vi "配置文件读取写入.vi"(7 "配置模式":enum16{"读取", "写入"}(ring), 8 "error in (no error)":errorcluster caption="错误输入（无错误）", 10 "配置文件名":string, 11 "配置信息":T6={"周期模式"=enum."不启用", "测量参数"={"氨氮"=TRUE, "总磷"=TRUE, "总氮"=TRUE, "CODMn"=TRUE, "CODCr"=FALSE}, "定点周期"={"启动命令"=enum."", "启动命令 2"=enum."", "启动命令 3"=enum."", "启动命令 4"=enum."", "启动命令 5"=enum."", "启动命令 6"=enum."", "启动命令 7"=enum."", "启动命令 8"=enum."", "启动命令 9"=enum."", "启动命令 10"=enum."", "启动命令 11"=enum."", "启动命令 12"=enum."", "启动命令 13"=enum."", "启动命令 14"=enum."", "启动命令 15"=enum."", "启动命令 16"=enum."", "启动命令 17"=enum."", "启动命令 18"=enum."", "启动命令 19"=enum."", "启动命令 20"=enum."", "启动命令 21"=enum."", "启动命令 22"=enum."", "启动命令 23"=enum."", "启动命令 24"=enum.""}, "间隔启动"={"启动命令"=enum."", "启动间隔"=0.0, "启动次数"=0}}) -> (0 "error out":errorcluster caption="错误输出", 3 "配置信息读取":T6={"周期模式"=enum."不启用", "测量参数"={"氨氮"=TRUE, "总磷"=TRUE, "总氮"=TRUE, "CODMn"=TRUE, "CODCr"=FALSE}, "定点周期"={"启动命令"=enum."", "启动命令 2"=enum."", "启动命令 3"=enum."", "启动命令 4"=enum."", "启动命令 5"=enum."", "启动命令 6"=enum."", "启动命令 7"=enum."", "启动命令 8"=enum."", "启动命令 9"=enum."", "启动命令 10"=enum."", "启动命令 11"=enum."", "启动命令 12"=enum."", "启动命令 13"=enum."", "启动命令 14"=enum."", "启动命令 15"=enum."", "启动命令 16"=enum."", "启动命令 17"=enum."", "启动命令 18"=enum."", "启动命令 19"=enum."", "启动命令 20"=enum."", "启动命令 21"=enum."", "启动命令 22"=enum."", "启动命令 23"=enum."", "启动命令 24"=enum.""}, "间隔启动"={"启动命令"=enum."", "启动间隔"=0.0, "启动次数"=0}})   [LabVIEW 2016, in "ZK定时设置.xctl"]
uses:
  <vilib>/Utility/xml.llb/Read From XML File(string).vi
  <vilib>/Utility/xml.llb/Write to XML File(string).vi
panel:
  # "分钟"
  # "次"
  # "分钟"
  # "次"
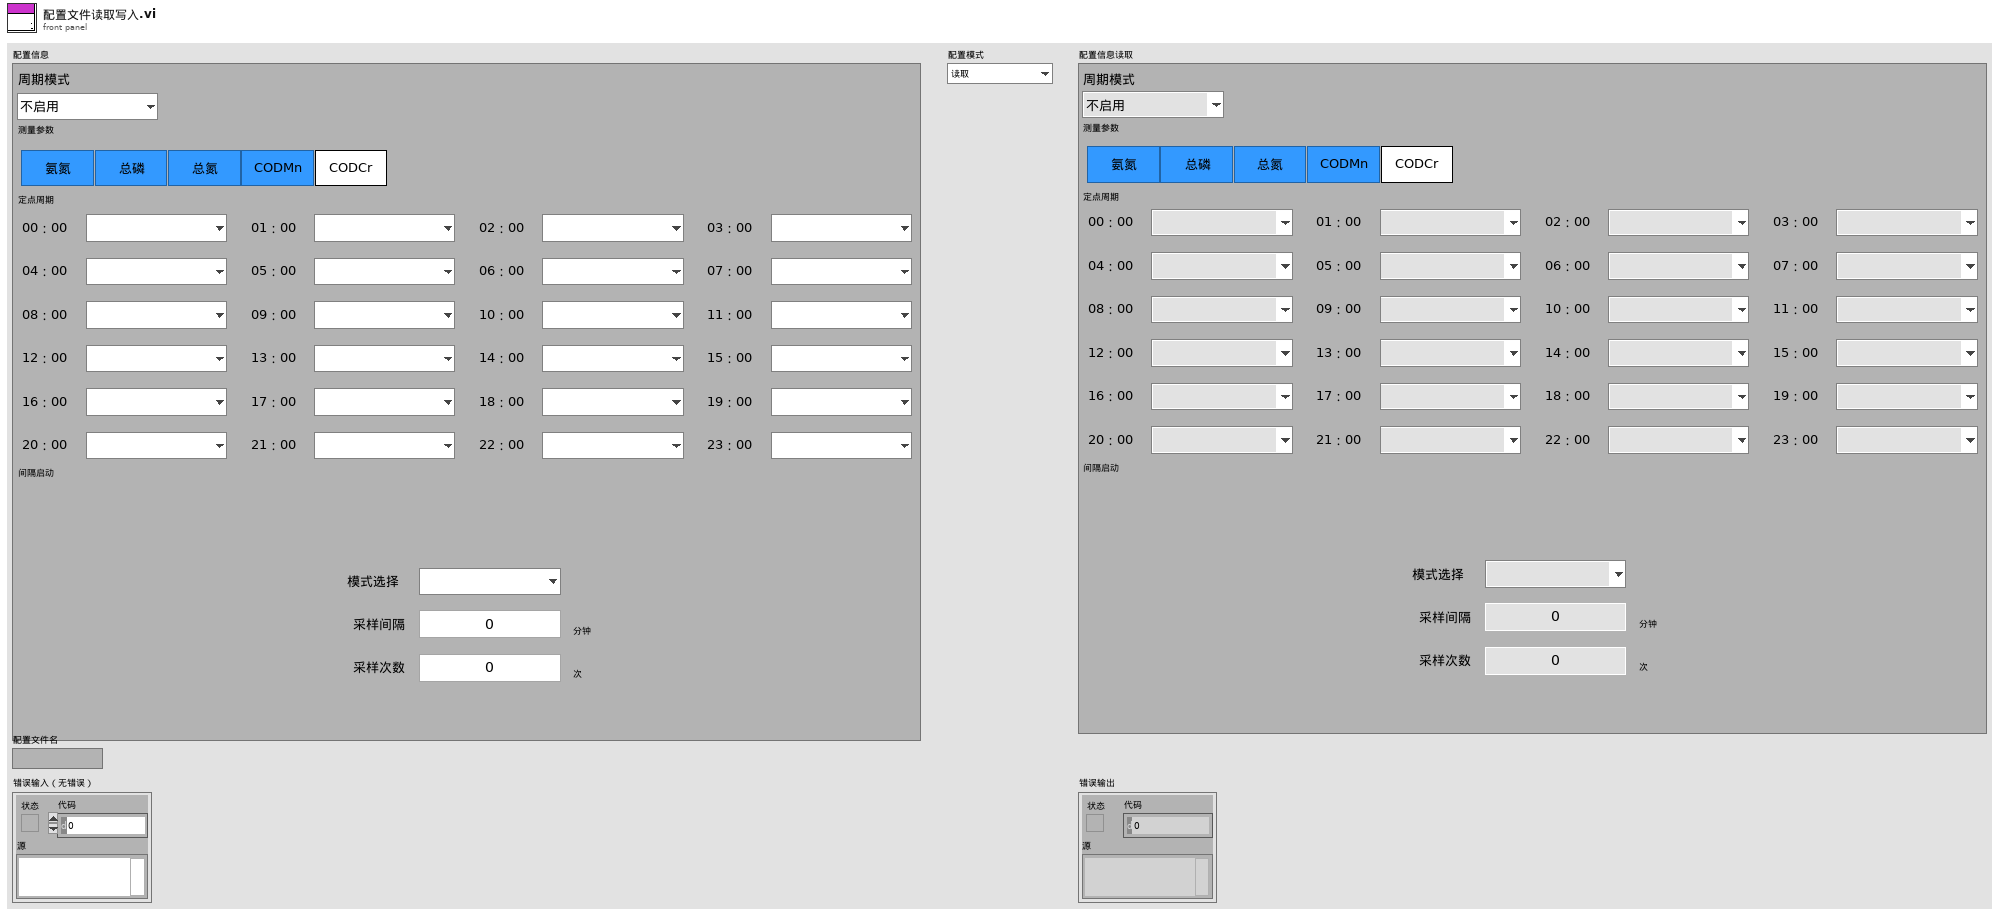
[diagram p1: front panel]
types:
  T1 = typedef "ZK定时设置.xctl/周期模式设置.ctl" = enum16{"不启用", "定点模式", "间隔模式"}
  T2 = typedef "ZK定时设置.xctl/测量参数.ctl" = cluster{"氨氮":bool, "总磷":bool, "总氮":bool, "CODMn":bool, "CODCr":bool}
  T3 = typedef "ZK定时设置.xctl/定点周期设置.ctl" = cluster{"启动命令":T4, "启动命令 2":T4, "启动命令 3":T4, "启动命令 4":T4, "启动命令 5":T4, "启动命令 6":T4, "启动命令 7":T4, "启动命令 8":T4, "启动命令 9":T4, "启动命令 10":T4, "启动命令 11":T4, "启动命令 12":T4, "启动命令 13":T4, "启动命令 14":T4, "启动命令 15":T4, "启动命令 16":T4, "启动命令 17":T4, "启动命令 18":T4, "启动命令 19":T4, "启动命令 20":T4, "启动命令 21":T4, "启动命令 22":T4, "启动命令 23":T4, "启动命令 24":T4}
  T4 = typedef "ZK定时设置.xctl/启动命令选择.ctl" = enum16{"", "加标回收（启动采配水）", "加标回收（不启动采配水）", "水样测试（启动采配水）", "水样测试（不启动采配水）", "平行样测试（启动采配水）", "平行样测试（不启动采配水）", "集成干预测试"}
  T5 = typedef "ZK定时设置.xctl/间隔启动设置.ctl" = cluster{"启动命令":T4, "启动间隔":dbl, "启动次数":i32}
  T6 = cluster{"周期模式":T1, "测量参数":T2, "定点周期":T3, "间隔启动":T5}
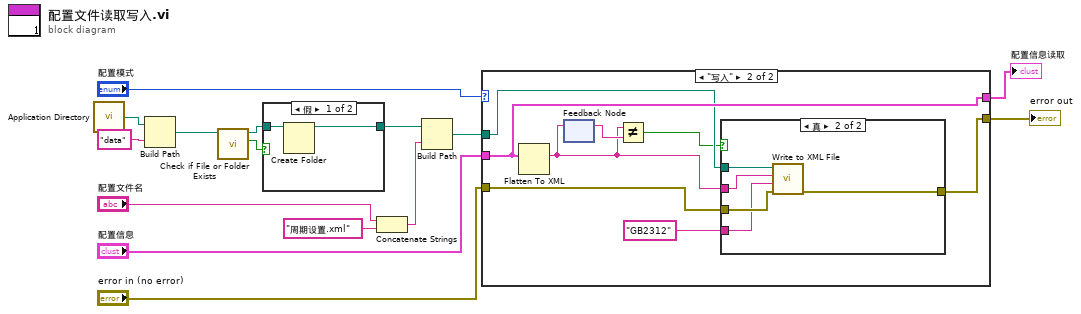
[diagram p0: block diagram]
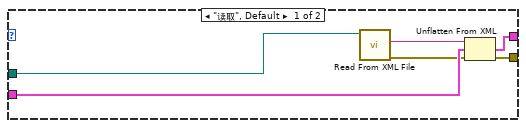
[diagram p2: hidden frame]
diagram:
  n1 = call <vilib>:"Application Directory.vi"() -> ("Application Directory"=w15:path)
  n2 = Build Path(base path=w15, name or relative path="data" ("名称或相对路径")) -> (appended path=w13:path)
  n3 = call <vilib>:"Check if File or Folder Exists.vi"("path"=w13) -> ("file or folder exists?"=w11:bool, "dup path"=w12:path)  [unwired: 8 in, 1 out]
  n4 = case shown="假" w11 {
    tunnel: w12 -> [w17 w18]
    tunnel: [w16 w18] -> w10
    frame False {
      n5 = Create Folder(path (use dialog)=w17) -> (created path=w16:path)  [unwired: 2 in, 2 out]
    }
    frame True {
    }
  }
  n6 = Concatenate Strings("配置文件名", "周期设置.xml" ("字符串")) -> (w8:string)
  n7 = Build Path(base path=w10, name or relative path=w8) -> (appended path=w3:path)
  n8 = case shown="\"写入\"" "配置模式" {
    tunnel: "配置信息" -> [w22 w32]
    tunnel: [w20 w28] -> w1
    tunnel: [w21 w32] -> w4
    tunnel: w3 -> [w24 w31]
    tunnel: "error in (no error)" -> [_ w30]
    frame "读取", Default {
      n9 = call-poly <vilib>:"Read From XML File.vi"("XML File Path"=w24) -> ("error out"=w19:errorcluster, "XML Elements"=w23:string)  [unwired: 8 in, 1 out]
      n10 = Unflatten From XML(xml string=w23, type=w22, error in (no error)=w19) -> (value=w21:T6, error out=w20:errorcluster)
    }
    frame "写入" {
      n11 = Flatten To XML(anything=w32) -> (xml string=w26:string)
      n12 = feedback-in #1(w26) -> ()
      n13 = feedback #1() -> (w27:string)  [unwired: 1 in]
      n14 = Not Equal?(x=w26, y=w27) -> (x != y?=w25:bool)
      n15 = case shown="真" w25 {
        tunnel: w31 -> [_ w38]
        tunnel: w30 -> [w33 w37]
        tunnel: "GB2312" ("XML Encoding") -> [_ w36]
        tunnel: [w33 w35] -> w28
        tunnel: w26 -> [_ w34]
        frame False {
        }
        frame True {
          n16 = call-poly <vilib>:"Write to XML File.vi"("error in (no error)"=w37, "XML Encoding"=w36, "XML Input"=w34, "XML File Path"=w38) -> ("error out"=w35:errorcluster)  [unwired: 5 in, 2 out]
        }
      }
    }
  }
  "配置信息读取" <- w4
  "error out" <- w1
